vi "Add Symbol Notification.vi"(7 "Alias":string, 8 "error in (no error)":errorcluster, 9 "Cycle Time (ms)":i32=60, 10 "Symbol Name":string, 11 "TwinCAT ADS in":refnum<class "TwinCAT ADS.lvclass">) -> (0 "error out":errorcluster, 3 "TwinCAT ADS out":refnum<class "TwinCAT ADS.lvclass">)   [LabVIEW 2018, in "TwinCAT ADS.lvclass"]
uses:
  TwinCAT ADS.lvclass
  Controls/Notifcation Map Value.ctl
  TwinCAT ADS.lvclass/TwinCAT ADS.ctl
  TwinCAT.Ads
  Get From Symbol Map.vi
  Get From Symbol Map Daemon.vi
  Get Notification Map.vi
  To Notification Key.vi
  Get Symbol Map.vi
  Format String.vi
  <vilib>/Utility/error.llb/Trim Whitespace.vi
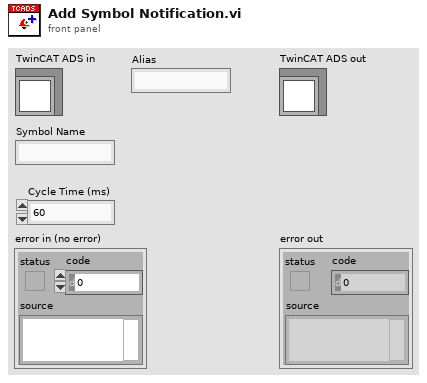
[diagram p1: front panel]
types:
  T1 = typedef "TwinCAT ADS.lvclass/Notifcation Map Value.ctl" = cluster{"Handle":i32, "Cycle Time":i32}
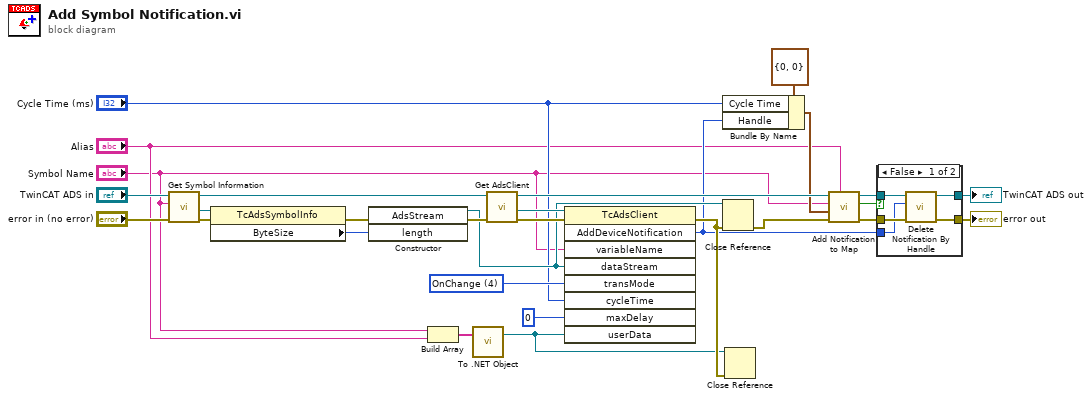
[diagram p0: block diagram]
diagram:
  w25 = 4 items=["None"=0, "ClientCycle"=1, "ClientOnChange"=2, "Cyclic"=3, "OnChange"=4, "CyclicInContext"=5, "OnChangeInContext"=6, "Client1Req"=10, "CyclicC0"=16, "CyclicC1"=17, "CyclicC2"=18, "CyclicC3"=19, "CyclicC4"=20, "CyclicC5"=21, "CyclicC6"=22, "CyclicC7"=23, "CyclicC8"=24, "CyclicC9"=25, "CyclicC10"=26, "CyclicC11"=27, "CyclicC12"=28, "CyclicC13"=29, "CyclicC14"=30, "CyclicC15"=31] ("transMode")
  n1 = call "Get Symbol Information.vi"("error in (no error)"="error in (no error)", "Symbol Name"="Symbol Name", "TwinCAT ADS in"="TwinCAT ADS in") -> ("error out"=w9:errorcluster, ".NET Symbol Information"=w5:refnum<k24>, "TwinCAT ADS out"=w7:refnum<class "TwinCAT ADS.lvclass">)  [unwired: 6 in]
  n2 = property class="TcAdsSymbolInfo"(reference=w5, error in=w9) -> (error out=w20:errorcluster, "ByteSize"=w18:i32)  [unwired: 1 out]
  n3 = constructor class="AdsStream"(error in=w20, "length"=w18) -> (reference out=w21:refnum<k24>, error out=w24:errorcluster)  [unwired: 2 in, 2 out]
  n4 = Build Array("Symbol Name", "Alias") -> (w1:string[])
  n5 = call <vilib>:"To .NET Object.vi"("anything"=w1) -> (".NET object"=w4:refnum<k24>)  [unwired: 1 in, 1 out]
  n6 = call "Get AdsClient.vi"("error in (no error)"=w24, "TwinCAT ADS in"=w7) -> ("error out"=w28:errorcluster, ".NET TcAdsClient"=w27:refnum<k24>, "TwinCAT ADS out"=w22:refnum<class "TwinCAT ADS.lvclass">)  [unwired: 7 in]
  n7 = invoke class="TcAdsClient" method="AddDeviceNotification"(reference=w27, error in=w28, "variableName"="Symbol Name", "dataStream"=w21, "transMode"=w25, "cycleTime"="Cycle Time (ms)", "maxDelay"=0, "userData"=w4) -> (error out=w29:errorcluster, "AddDeviceNotification"=w10:i32)  [unwired: 1 in, 7 out]
  n8 = Bundle By Name(cluster=T1 {"Handle"=0, "Cycle Time"=0} ("Value"), "Cycle Time"="Cycle Time (ms)", "Handle"=w10) -> (w16:T1)
  n9 = Close Reference(reference=w21, error in (no error)=w29) -> (error out=w17:errorcluster)
  n10 = Close Reference(reference=w4, error in (no error)=w29) -> ()  [unwired: 1 out]
  n11 = call "Add Notification to Map.vi"("Alias"="Alias", "error in (no error)"=w17, "Value"=w16, "Symbol Name"="Symbol Name", "TwinCAT ADS in"=w22) -> ("error out"=w14:errorcluster, "Success?"=w11:bool, "TwinCAT ADS out"=w15:refnum<class "TwinCAT ADS.lvclass">)  [unwired: 4 in]
  n12 = case shown="False" w11 {
    tunnel: w15 -> [w34 w36]
    tunnel: w14 -> [w33 w35]
    tunnel: [w32 w35] -> w13
    tunnel: [w31 w36] -> w12
    tunnel: w10 -> [w30 _]
    frame False {
      n13 = call "Delete Notification By Handle.vi"("error in (no error)"=w33, "Handle"=w30, "TwinCAT ADS in"=w34) -> ("error out"=w32:errorcluster, "TwinCAT ADS out"=w31:refnum<class "TwinCAT ADS.lvclass">)  [unwired: 7 in]
    }
    frame True {
    }
  }
  "error out" <- w13
  "TwinCAT ADS out" <- w12
